vi "05.1 Average.vi"() -> ()   [LabVIEW 2019]
panel:
  out "Average":dbl
  in  "X5":sgl
  in  "X4":sgl
  in  "X3":sgl
  in  "X2":sgl
  in  "X1":sgl
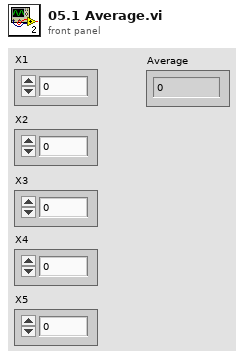
[diagram p1: front panel]
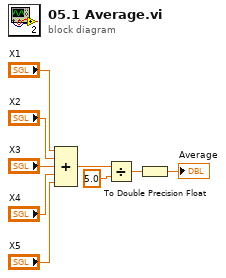
[diagram p0: block diagram]
diagram:
  n1 = Compound Arithmetic op=ADD("X1", "X2", "X3", "X4", "X5") -> (w3:sgl)
  n2 = Divide(x=w3, y=sgl 5.0) -> (x/y=w2:sgl)
  n3 = To Double Precision Float(number=w2) -> (double precision float=→"Average":dbl)
